vi "Wait.Gui.Init.vi"(8 "error in (no error)":errorcluster) -> (0 "error out":errorcluster)   [LabVIEW 2016]
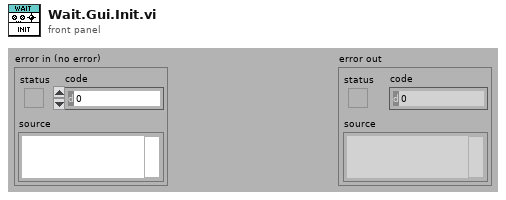
[diagram p1: front panel]
types:
  T1 = enum32{"Invalid", "Standard", "Closed", "Hidden", "Minimized", "Maximized"}
  T2 = enum32{"Bad", "Idle", "Run top level", "Running"}
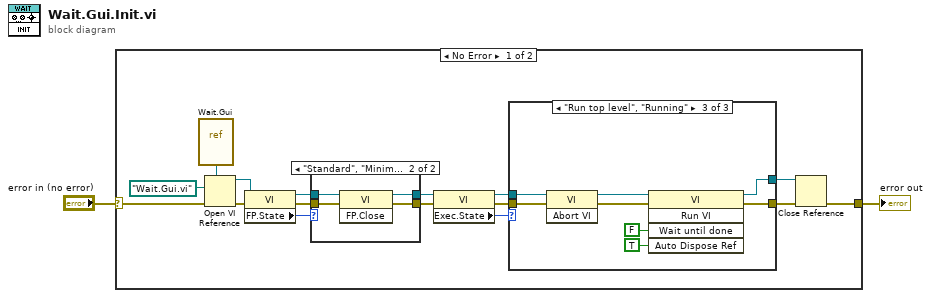
[diagram p0: block diagram]
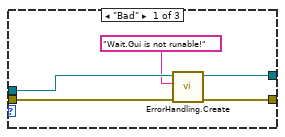
[diagram p3: hidden frame]
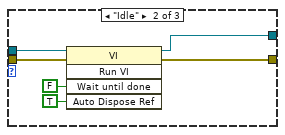
[diagram p4: hidden frame]
diagram:
  n1 = case shown="No Error" "error in (no error)" {
    selector: "error in (no error)" -> [w16 w43]
    tunnel: [w15 w43] -> w2
    frame No Error {
      n2 = vi-ref "Wait.Gui.vi"() -> (w18:refnum<vi>)
      n3 = Open VI Reference(type specifier VI Refnum (for type only)=w18, vi path=path "Wait.Gui.vi", error in (no error)=w16) -> (vi reference=w5:refnum<vi>, error out=w6:errorcluster)  [unwired: 3 in]
      n4 = property class="VI"(reference=w5, error in=w6) -> (reference out=w7:refnum<vi>, error out=w9:errorcluster, "FP.State"=w8:T1)
      n5 = case shown="\"Standard\", \"Minimized\", \"Maximized\"" w8 {
        tunnel: [w19 w24] -> w11
        tunnel: [w20 w23] -> w10
        tunnel: w9 -> [w19 w22]
        tunnel: w7 -> [w20 w21]
        frame Default {
        }
        frame "Standard", "Minimized", "Maximized" {
          n6 = invoke class="VI" method="FP.Close"(reference=w21, error in=w22) -> (reference out=w23:refnum<vi>, error out=w24:errorcluster)  [unwired: 1 in, 1 out]
        }
      }
      n7 = property class="VI"(reference=w10, error in=w11) -> (reference out=w12:refnum<vi>, error out=w13:errorcluster, "Exec.State"=w14:T2)
      n8 = case shown="\"Run top level\", \"Running\"" w14 {
        tunnel: [w26 w33 w36] -> w4
        tunnel: w13 -> [w27 w31 w40]
        tunnel: [w28 w32 w35] -> w3
        tunnel: w12 -> [w28 w34 w39]
        frame "Bad" {
          n9 = call "ErrorHandling.Create.vi"("error in"=w27, "explanation"="Wait.Gui is not runable!") -> ("error out"=w26:errorcluster)  [unwired: 9 in]
        }
        frame "Idle" {
          n10 = invoke class="VI" method="Run VI"(reference=w34, error in=w31, "Wait until done"=FALSE ("Wait Until Done"), "Auto Dispose Ref"=TRUE ("Auto Dispose Reference")) -> (reference out=w32:refnum<vi>, error out=w33:errorcluster)  [unwired: 1 in, 3 out]
        }
        frame "Run top level", "Running" {
          n11 = invoke class="VI" method="Abort VI"(reference=w39, error in=w40) -> (reference out=w37:refnum<vi>, error out=w38:errorcluster)  [unwired: 1 in, 1 out]
          n12 = invoke class="VI" method="Run VI"(reference=w37, error in=w38, "Wait until done"=FALSE ("Wait Until Done"), "Auto Dispose Ref"=TRUE ("Auto Dispose Reference")) -> (reference out=w35:refnum<vi>, error out=w36:errorcluster)  [unwired: 1 in, 3 out]
        }
      }
      n13 = Close Reference(reference=w3, error in (no error)=w4) -> (error out=w15:errorcluster)
    }
    frame Error {
    }
  }
  "error out" <- w2
